vi "KepcoDCPwr transient.vi"(0 "VISA Session":refnum<visa-resource-name>, 1 "Mode":bool, 5 "Model In":string, 7 "channel name (\"\")":string="\"\"", 9 "Trans Enabled":bool caption="Transient enabled (True)", 11 "error in (no error)":errorcluster {"code" format="%.0x"}, 12 "Trans Time":dbl, 13 "Trans Value":dbl) -> (4 "VISA Session Out":refnum<visa-resource-name>, 6 "Model Out":string, 8 "channel name out (\"\")":string="\"\"" caption="channel name Out (\"\")", 15 "error out":errorcluster {"code" format="%.0x"})   [LabVIEW 2013]
doc: "Configures whether the signal that the power supply produces on a channel appears at the output connector."
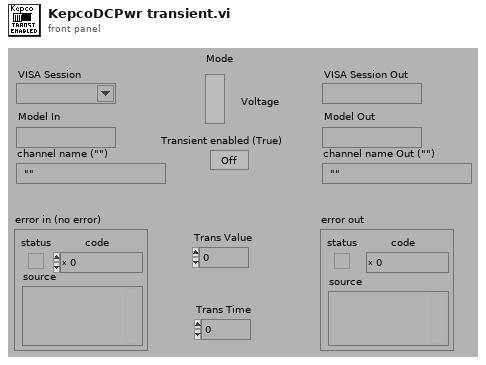
[diagram p1: front panel]
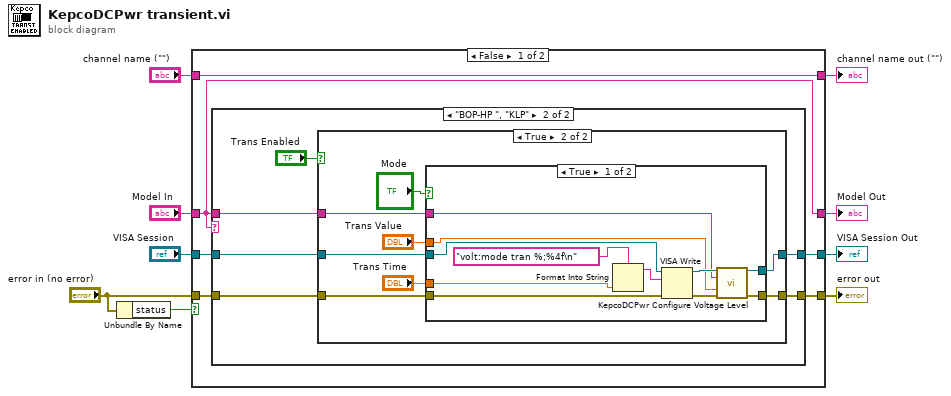
[diagram p0: block diagram]
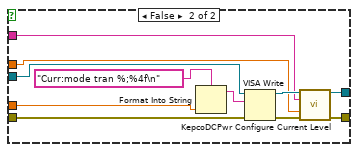
[diagram p4: hidden frame]
diagram:
  n1 = Unbundle By Name("error in (no error)") -> ("status"=w7:bool)
  n2 = case shown="False" w7 {
    tunnel: [w14 w59] -> w9
    tunnel: "error in (no error)" -> [w13 w59]
    tunnel: [w15 w58] -> w6
    tunnel: "VISA Session" -> [w12 w58]
    tunnel: "Model In" -> [w10 w57]
    tunnel: [w10 w57] -> w3
    tunnel: "channel name (\"\")" -> [w11 w56]
    tunnel: [w11 w56] -> w1
    frame False {
      n3 = case shown="\"BOP-HP \", \"KLP\"" w10 {
        tunnel: [w16 w23] -> w15
        tunnel: [w17 w22] -> w14
        tunnel: w13 -> [w17 w20]
        tunnel: w12 -> [w16 w19]
        tunnel: w10 -> [_ w18]
        frame "False", Default {
        }
        frame "BOP-HP ", "KLP" {
          n4 = case shown="True" "Trans Enabled" {
            tunnel: w19 -> [w24 w33]
            tunnel: [w25 w30] -> w22
            tunnel: [w24 w31] -> w23
            tunnel: w20 -> [w25 w32]
            tunnel: w18 -> [_ w29]
            frame False {
            }
            frame True {
              n5 = case shown="True" "Mode" {
                tunnel: w33 -> [w44 w55]
                tunnel: w32 -> [w43 w54]
                tunnel: [w41 w52] -> w31
                tunnel: [w40 w51] -> w30
                tunnel: w29 -> [w38 w49]
                tunnel: "Trans Time" -> [w35 w46]
                tunnel: "Trans Value" -> [w34 w45]
                frame True {
                  n6 = Format Into String(format string="volt:mode tran %;%4f\n", w35) -> (resulting string=w36:string)  [unwired: 2 in, 1 out]
                  n7 = VISA Write(VISA resource name=w44, write buffer=w36, error in (no error)=w43) -> (VISA resource name out=w42:refnum<visa-resource-name>, error out=w39:errorcluster)  [unwired: 1 out]
                  n8 = call "KepcoDCPwr Configure Voltage Level.vi"("VISA Session"=w42, "Model In"=w38, "level (0.0 volts)"=w34, "error in (no error)"=w39) -> ("VISA Session Out"=w41:refnum<visa-resource-name>, "error out"=w40:errorcluster)  [unwired: 8 in, 2 out]
                }
                frame False {
                  n9 = Format Into String(format string="Curr:mode tran %;%4f\n", w46) -> (resulting string=w47:string)  [unwired: 2 in, 1 out]
                  n10 = VISA Write(VISA resource name=w55, write buffer=w47, error in (no error)=w54) -> (VISA resource name out=w53:refnum<visa-resource-name>, error out=w50:errorcluster)  [unwired: 1 out]
                  n11 = call "KepcoDCPwr Configure Current Level.vi"("VISA Session"=w53, "Model In"=w49, "level (0.0 volts)"=w45, "error in (no error)"=w50) -> ("VISA Session Out"=w52:refnum<visa-resource-name>, "error out"=w51:errorcluster)  [unwired: 8 in, 2 out]
                }
              }
            }
          }
        }
      }
    }
    frame True {
    }
  }
  "error out" <- w9
  "VISA Session Out" <- w6
  "Model Out" <- w3
  "channel name out (\"\")" <- w1
